vi "Main VI.vi"() -> ()   [LabVIEW 2016, in "Drona basic.lvlib"]
doc: "This VI performs the operation of basic drona, getting the active VI, populating the right click of control with Drona and also getting the drona path of the value changed control"
uses:
  Drona basic.lvlib
  Typedefs/Data.ctl
  <vilib>/SLL Toolkit/SLL Queued State Machine/Queue Driver/Typedefs/Queue Type.ctl
  Typedefs/cluster array.ctl
  <vilib>/Utility/miscctls.llb/LVPoint32TypeDef.ctl
  <vilib>/SLL Toolkit/SLL Queued State Machine/Queue Driver/Create Queue.vi
  <vilib>/SLL Toolkit/SLL Queued State Machine/Queue Driver/Enqueue an Item to Queue.vi
  <vilib>/SLL Toolkit/SLL Queued State Machine/Queue Driver/Dequeue Queue.vi
  <vilib>/SLL Toolkit/SLL Queued State Machine/Queue Driver/Enqueue N Items.vi
  <vilib>/SLL Toolkit/SLL Queued State Machine/Queue Driver/Flush Queue.vi
  <vilib>/SLL Toolkit/SLL Queued State Machine/Queue Driver/Release Queue.vi
  <vilib>/SLL Toolkit/SLL Queued State Machine/SLL QSM.lvlib
panel:
  out "Event and Drona Path:":string
  out "Error Out":errorcluster
  in  "Error In":errorcluster
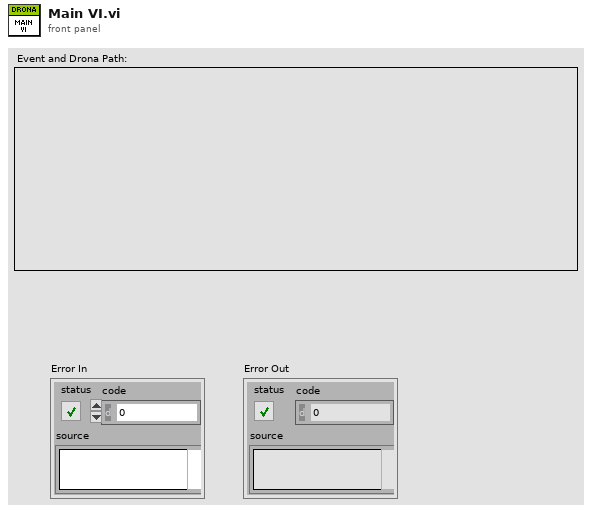
[diagram p1: front panel]
types:
  T1 = typedef "Drona basic.lvlib/Data.ctl" = cluster{"AppRef":refnum<vi>, "Active VIName":string, "Queue Ref":refnum<queue>, "ActiveVI reference":refnum<vi>, "Cluster references":refnum<vi>[], "Control References":refnum<vi>[], "Drona path,ref":T2[], "SelList ":refnum<vi>[], "Drona name":string, "Panes event refnum":refnum<event-registration>, "MenuRef":refnum<k9>, "Controls event refnum":refnum<event-registration>, "CtlRef":refnum<vi>, "Control name":string, "NewVal":variant, "OldVal":variant, "Point32":T3, "Ref array":refnum<vi>[], "Event ":string, "Event Registration Refnum ":refnum<event-registration>, "Subpanel reference":refnum<vi>, "Inserted VI ref":refnum<vi>, "SP Ref array":refnum<vi>[], "SP Registration Refnum":refnum<event-registration>, "User Events":cluster{"Panes event refnum":refnum<event-registration>, "Event Registration Refnum ":refnum<event-registration>, "SP Registration Refnum":refnum<event-registration>}}
  T2 = typedef "Drona basic.lvlib/cluster array.ctl" = cluster{"Control name":string, "Control reference":refnum<vi>}
  T3 = typedef "LVPoint32TypeDef.ctl" = cluster{"Horizontal":i32, "Vertical":i32}
  T4 = cluster{"Panes event refnum":refnum<event-registration>, "Event Registration Refnum ":refnum<event-registration>, "SP Registration Refnum":refnum<event-registration>}
  T5 = enum32{"Bad", "Idle", "Run top level", "Running"}
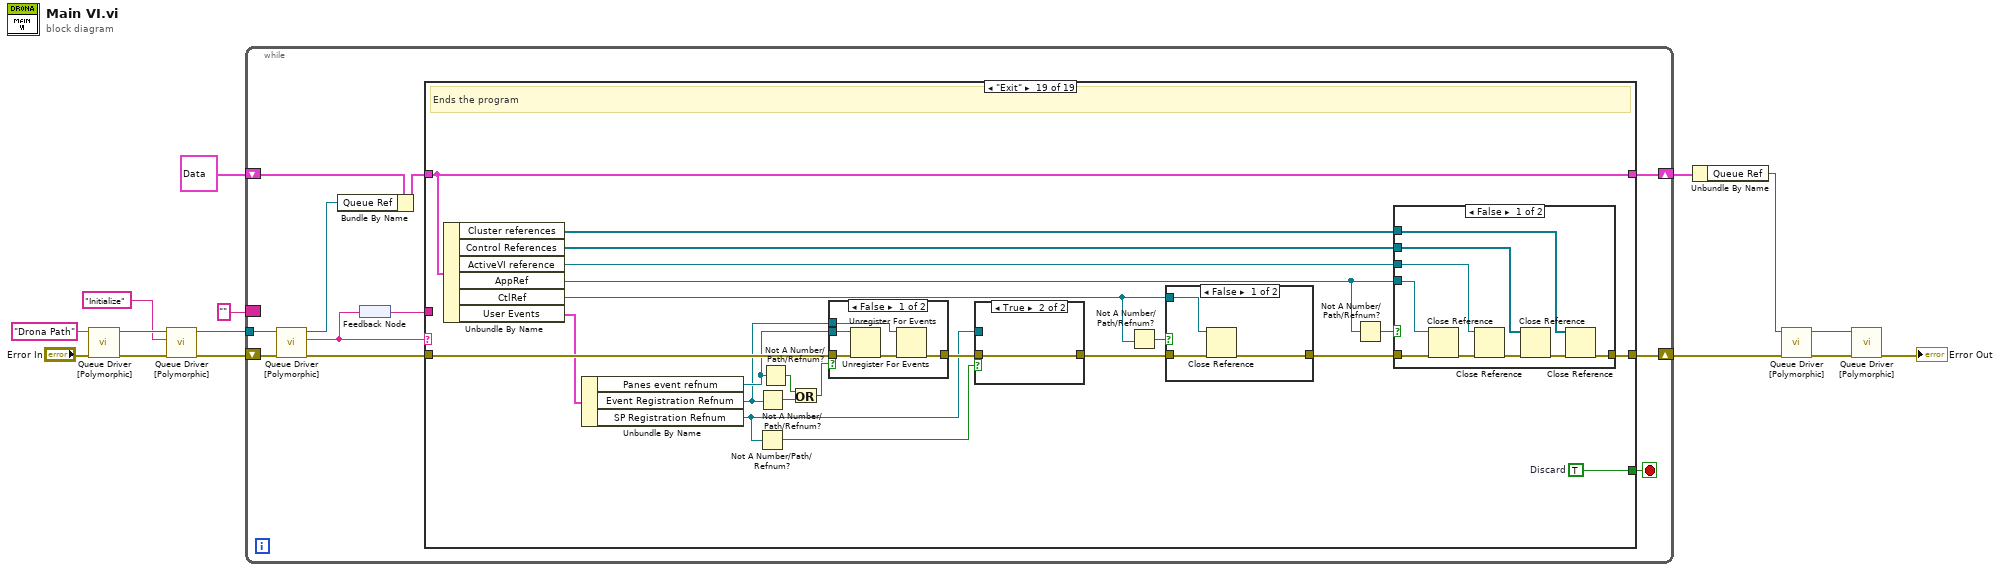
[diagram p0: block diagram]
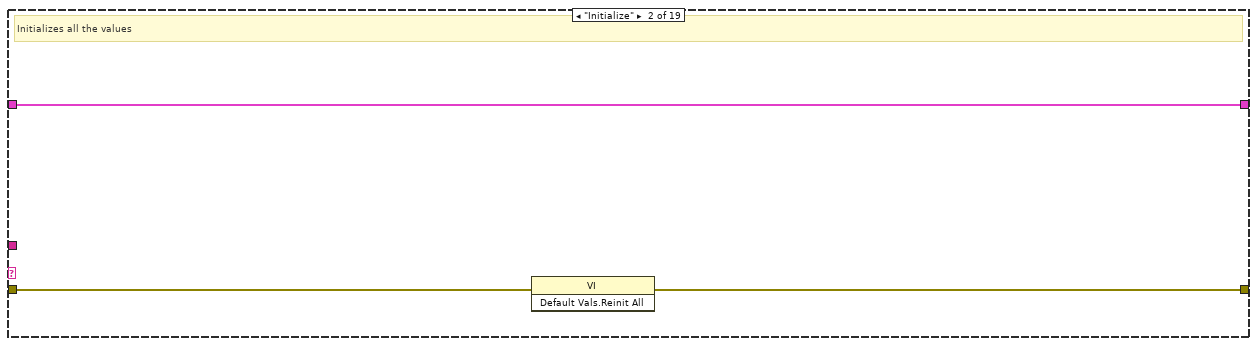
[diagram p3: hidden frame]
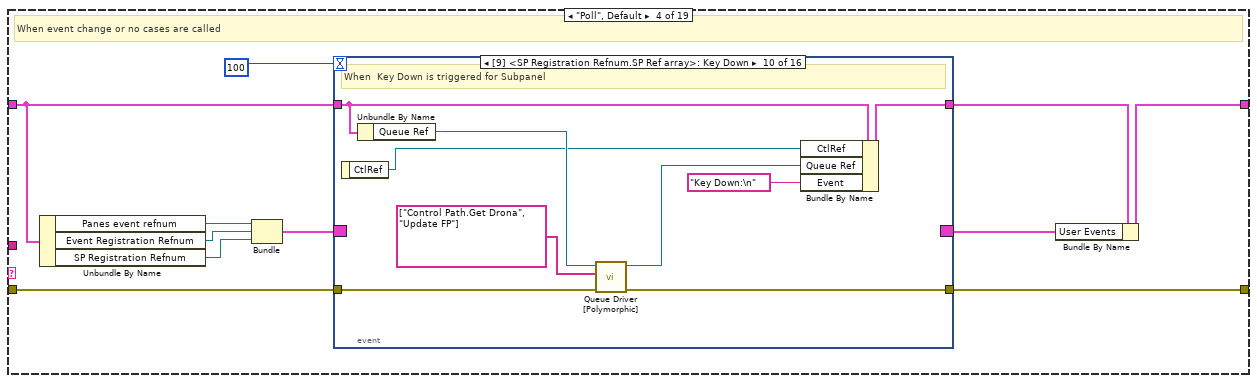
[diagram p5: hidden frame]
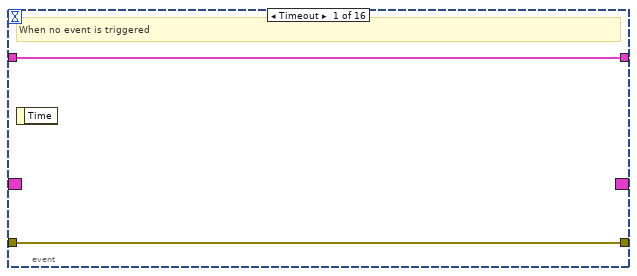
[diagram p6: hidden frame]
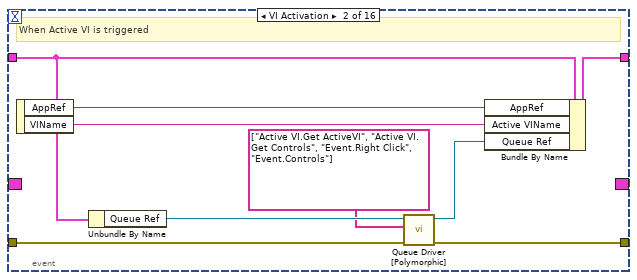
[diagram p7: hidden frame]
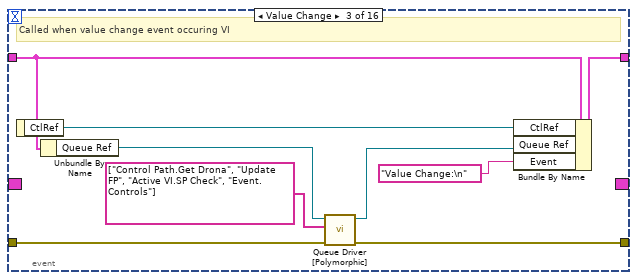
[diagram p8: hidden frame]
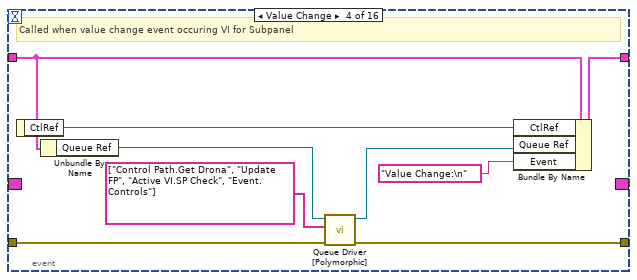
[diagram p9: hidden frame]
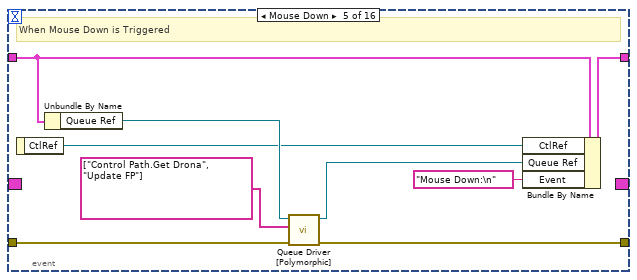
[diagram p10: hidden frame]
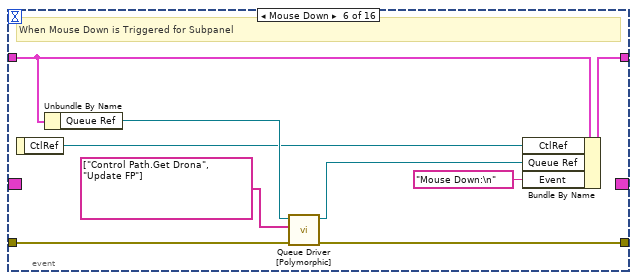
[diagram p11: hidden frame]
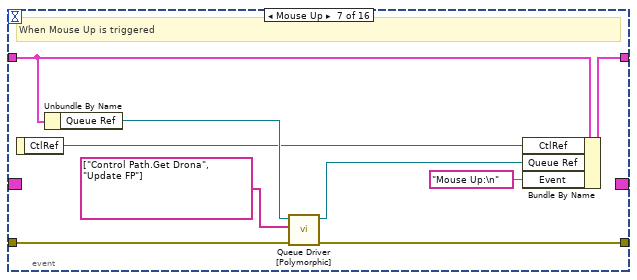
[diagram p12: hidden frame]
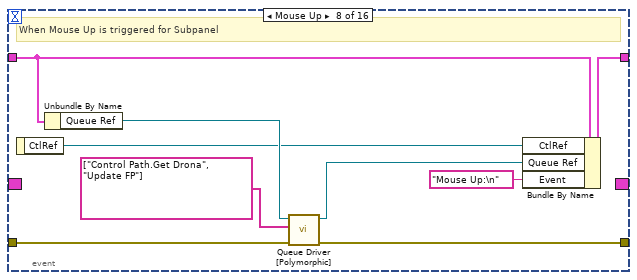
[diagram p13: hidden frame]
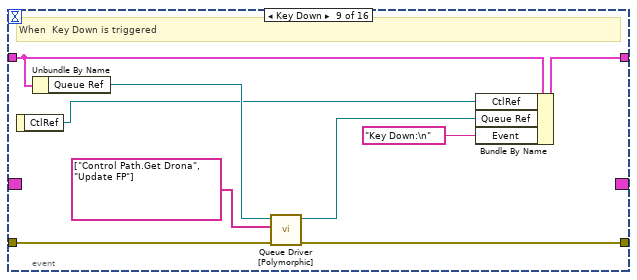
[diagram p14: hidden frame]
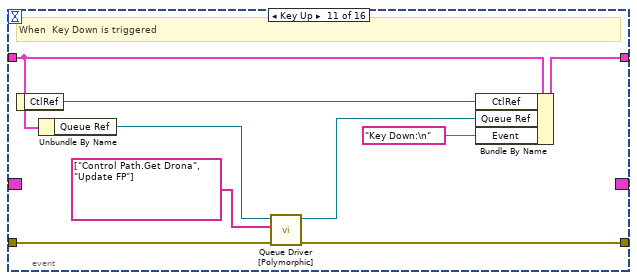
[diagram p15: hidden frame]
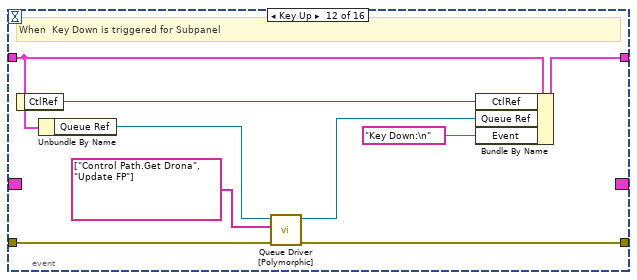
[diagram p16: hidden frame]
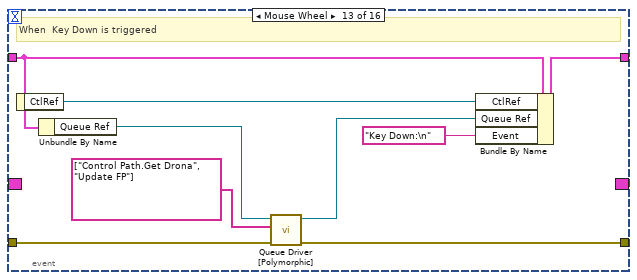
[diagram p17: hidden frame]
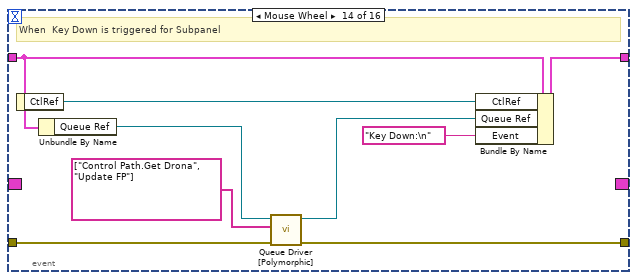
[diagram p18: hidden frame]
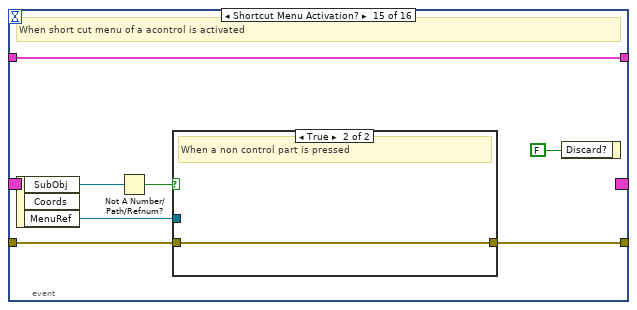
[diagram p19: hidden frame]
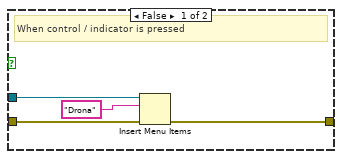
[diagram p20: hidden frame]
diagram:
  n1 = call-poly <vilib>:"Queue Driver [Polymorphic].vi"("Error In"="Error In", "Queue Name (Optional)"="Drona Path") -> ("Error Out"=w14:errorcluster, "Queue Ref"=w12:refnum<queue>)  [unwired: 8 in]
  n2 = call-poly <vilib>:"Queue Driver [Polymorphic].vi"("Error In"=w14, "Item to Add"="Initialize", "Queue Ref In"=w12) -> ("Error Out"=w9:errorcluster, "Queue Ref Out"=w8:refnum<queue>)  [unwired: 7 in]
  n3 = while {
    shift-right: [w26] -> w6
    shift-left: T1 {"AppRef"=refnum, "Active VIName"="", "Queue Ref"=refnum, "ActiveVI reference"=refnum, "Cluster references"=[], "Control References"=[], "Drona path,ref"=[], "SelList "=[], "Drona name"="", "Panes event refnum"=refnum, "MenuRef"=refnum, "Controls event refnum"=refnum, "CtlRef"=refnum, "Control name"="", "NewVal"=variant, "OldVal"=variant, "Point32"={"Horizontal"=0, "Vertical"=0}, "Ref array"=[], "Event "="", "Event Registration Refnum "=refnum, "Subpanel reference"=refnum, "Inserted VI ref"=refnum, "SP Ref array"=[], "SP Registration Refnum"=refnum, "User Events"={"Panes event refnum"=refnum, "Event Registration Refnum "=refnum, "SP Registration Refnum"=refnum}} -> [w23]
    tunnel: w8 -> [w24]
    shift-right: [w20] -> w7
    shift-left: w9 -> [w25]
    border: "" ("Feedback constant") -> [_]
    stop <- w18 stop-if-true
    n4 = call-poly <vilib>:"Queue Driver [Polymorphic].vi"("Error In"=w25, "Queue Ref In"=w24) -> ("Error Out"=w19:errorcluster, "Dequeue"=w17:string, "Queue Ref Out"=w21:refnum<queue>)  [unwired: 6 in, 1 out]
    n5 = Bundle By Name(cluster=w23, "Queue Ref"=w21) -> (w22:T1)
    n6 = feedback-in #1(w17) -> ()
    n7 = feedback #1() -> (w16:string)
    n8 = case shown="\"Exit\"" w17 {
      tunnel: [w28 w31 w33 w35 w185 w188 w190 w200 w221 w296 w319 w334 w356 w363 w370 w377 w380 w402 w423] -> w26
      tunnel: w22 -> [w28 w31 w33 w41 w185 w188 w190 w201 w222 w297 w319 w333 w356 w364 w371 w377 w381 w402 w423]
      tunnel: [w27 w29 w32 w43 w186 w187 w189 w191 w224 w302 w318 w330 w355 w365 w372 w376 w383 w401 w422] -> w20
      tunnel: w19 -> [w27 w30 w32 w42 w186 w187 w189 w203 w223 w303 w318 w326 w355 w360 w367 w376 w392 w401 w413]
      tunnel: [_ _ _ _ _ _ _ _ _ _ _ _ _ _ _ _ _ _ w424] -> w18
      tunnel: w16 -> [_ _ _ _ _ _ _ _ _ _ _ _ _ _ _ _ w389 _ _]
      frame "<-----------Initialize---------->" {
      }
      frame "Initialize" {
        # "Initializes all the values"
        n9 = invoke class="VI" method="Default Vals.Reinit All"(error in=w30) -> (error out=w29:errorcluster)  [unwired: 2 in, 2 out]
      }
      frame "<------Front panel cases------>" {
      }
      frame "Poll", Default {
        # "When event change or no cases are called"
        n10 = Unbundle By Name(w41) -> ("Panes event refnum"=w40:refnum<event-registration>, "Event Registration Refnum"=w37:refnum<event-registration>, "SP Registration Refnum"=w36:refnum<event-registration>)
        n11 = Bundle("Panes event refnum"=w40, "Event Registration Refnum"=w37, "SP Registration Refnum"=w36) -> (w39:T4)  [unwired: 1 in]
        n12 = event shown="[9] <SP Registration Refnum.SP Ref array>: Key Down" {
          selector: w39 -> [_ _ _ _ _ _ _ _ _ _ _ _ _ _ _ _]
          dyn-events: [_ _ _ _ _ _ _ _ _ _ _ _ _ _ _ _] -> w34
          timeout: 100 -> [_ _ _ _ _ _ _ _ _ _ _ _ _ _ _ _]
          tunnel: [w46 w55 w64 w73 w81 w90 w99 w108 w112 w121 w130 w139 w148 w157 w164 w178] -> w38
          tunnel: w41 -> [w46 w50 w61 w70 w80 w89 w98 w107 w111 w120 w129 w138 w147 w156 w164 w179]
          tunnel: [w45 w51 w62 w71 w79 w88 w97 w106 w118 w127 w136 w145 w154 w163 w169 w182] -> w43
          tunnel: w42 -> [w45 w52 w63 w72 w82 w91 w100 w109 w117 w126 w135 w144 w153 w162 w170 w176]
          event Timeout {
            # "When no event is triggered"
            n13 = event-data() -> ()  [unwired: 1 in, 1 out]
          }
          event VI Activation {
            # "When Active VI is triggered"
            n14 = event-data() -> ("AppRef"=w54:refnum<vi>, "VIName"=w53:string)  [unwired: 1 in]
            n15 = Unbundle By Name(w50) -> ("Queue Ref"=w49:refnum<queue>)
            n16 = call-poly <vilib>:"Queue Driver [Polymorphic].vi"("Error In"=w52, "Enqueue N"=string[] ["Active VI.Get ActiveVI", "Active VI.Get Controls", "Event.Right Click", "Event.Controls"], "Queue Ref In"=w49) -> ("Error Out"=w51:errorcluster, "Queue Ref Out"=w48:refnum<queue>)  [unwired: 7 in]
            n17 = Bundle By Name(cluster=w50, "AppRef"=w54, "Active VIName"=w53, "Queue Ref"=w48) -> (w55:T1)
          }
          event Value Change {
            # "Called when value change event occuring VI"
            n18 = event-data() -> ("CtlRef"=w58:refnum<vi>)  [unwired: 1 in]
            n19 = Unbundle By Name(w61) -> ("Queue Ref"=w60:refnum<queue>)
            n20 = call-poly <vilib>:"Queue Driver [Polymorphic].vi"("Error In"=w63, "Enqueue N"=string[] ["Control Path.Get Drona", "Update FP", "Active VI.SP Check", "Event.Controls"], "Queue Ref In"=w60) -> ("Error Out"=w62:errorcluster, "Queue Ref Out"=w59:refnum<queue>)  [unwired: 7 in]
            n21 = Bundle By Name(cluster=w61, "CtlRef"=w58, "Queue Ref"=w59, "Event"="Value Change:\n") -> (w64:T1)
          }
          event Value Change {
            # "Called when value change event occuring VI for Subpanel"
            n22 = event-data() -> ("CtlRef"=w67:refnum<vi>)  [unwired: 1 in]
            n23 = Unbundle By Name(w70) -> ("Queue Ref"=w69:refnum<queue>)
            n24 = call-poly <vilib>:"Queue Driver [Polymorphic].vi"("Error In"=w72, "Enqueue N"=string[] ["Control Path.Get Drona", "Update FP", "Active VI.SP Check", "Event.Controls"], "Queue Ref In"=w69) -> ("Error Out"=w71:errorcluster, "Queue Ref Out"=w68:refnum<queue>)  [unwired: 7 in]
            n25 = Bundle By Name(cluster=w70, "CtlRef"=w67, "Queue Ref"=w68, "Event"="Value Change:\n") -> (w73:T1)
          }
          event Mouse Down {
            # "When Mouse Down is Triggered"
            n26 = event-data() -> ("CtlRef"=w76:refnum<vi>)  [unwired: 1 in]
            n27 = Unbundle By Name(w80) -> ("Queue Ref"=w78:refnum<queue>)
            n28 = call-poly <vilib>:"Queue Driver [Polymorphic].vi"("Error In"=w82, "Enqueue N"=string[] ["Control Path.Get Drona", "Update FP"], "Queue Ref In"=w78) -> ("Error Out"=w79:errorcluster, "Queue Ref Out"=w77:refnum<queue>)  [unwired: 7 in]
            n29 = Bundle By Name(cluster=w80, "CtlRef"=w76, "Queue Ref"=w77, "Event"="Mouse Down:\n") -> (w81:T1)
          }
          event Mouse Down {
            # "When Mouse Down is Triggered for Subpanel"
            n30 = event-data() -> ("CtlRef"=w85:refnum<vi>)  [unwired: 1 in]
            n31 = Unbundle By Name(w89) -> ("Queue Ref"=w87:refnum<queue>)
            n32 = call-poly <vilib>:"Queue Driver [Polymorphic].vi"("Error In"=w91, "Enqueue N"=string[] ["Control Path.Get Drona", "Update FP"], "Queue Ref In"=w87) -> ("Error Out"=w88:errorcluster, "Queue Ref Out"=w86:refnum<queue>)  [unwired: 7 in]
            n33 = Bundle By Name(cluster=w89, "CtlRef"=w85, "Queue Ref"=w86, "Event"="Mouse Down:\n") -> (w90:T1)
          }
          event Mouse Up {
            # "When Mouse Up is triggered"
            n34 = event-data() -> ("CtlRef"=w94:refnum<vi>)  [unwired: 1 in]
            n35 = Unbundle By Name(w98) -> ("Queue Ref"=w96:refnum<queue>)
            n36 = call-poly <vilib>:"Queue Driver [Polymorphic].vi"("Error In"=w100, "Enqueue N"=string[] ["Control Path.Get Drona", "Update FP"], "Queue Ref In"=w96) -> ("Error Out"=w97:errorcluster, "Queue Ref Out"=w95:refnum<queue>)  [unwired: 7 in]
            n37 = Bundle By Name(cluster=w98, "CtlRef"=w94, "Queue Ref"=w95, "Event"="Mouse Up:\n") -> (w99:T1)
          }
          event Mouse Up {
            # "When Mouse Up is triggered for Subpanel"
            n38 = event-data() -> ("CtlRef"=w103:refnum<vi>)  [unwired: 1 in]
            n39 = Unbundle By Name(w107) -> ("Queue Ref"=w105:refnum<queue>)
            n40 = call-poly <vilib>:"Queue Driver [Polymorphic].vi"("Error In"=w109, "Enqueue N"=string[] ["Control Path.Get Drona", "Update FP"], "Queue Ref In"=w105) -> ("Error Out"=w106:errorcluster, "Queue Ref Out"=w104:refnum<queue>)  [unwired: 7 in]
            n41 = Bundle By Name(cluster=w107, "CtlRef"=w103, "Queue Ref"=w104, "Event"="Mouse Up:\n") -> (w108:T1)
          }
          event Key Down {
            # "When  Key Down is triggered"
            n42 = event-data() -> ("CtlRef"=w114:refnum<vi>)  [unwired: 1 in]
            n43 = Unbundle By Name(w111) -> ("Queue Ref"=w116:refnum<queue>)
            n44 = call-poly <vilib>:"Queue Driver [Polymorphic].vi"("Error In"=w117, "Enqueue N"=string[] ["Control Path.Get Drona", "Update FP"], "Queue Ref In"=w116) -> ("Error Out"=w118:errorcluster, "Queue Ref Out"=w113:refnum<queue>)  [unwired: 7 in]
            n45 = Bundle By Name(cluster=w111, "CtlRef"=w114, "Queue Ref"=w113, "Event"="Key Down:\n") -> (w112:T1)
          }
          event Key Down {
            # "When  Key Down is triggered for Subpanel"
            n46 = event-data() -> ("CtlRef"=w123:refnum<vi>)  [unwired: 1 in]
            n47 = Unbundle By Name(w120) -> ("Queue Ref"=w125:refnum<queue>)
            n48 = call-poly <vilib>:"Queue Driver [Polymorphic].vi"("Error In"=w126, "Enqueue N"=string[] ["Control Path.Get Drona", "Update FP"], "Queue Ref In"=w125) -> ("Error Out"=w127:errorcluster, "Queue Ref Out"=w122:refnum<queue>)  [unwired: 7 in]
            n49 = Bundle By Name(cluster=w120, "CtlRef"=w123, "Queue Ref"=w122, "Event"="Key Down:\n") -> (w121:T1)
          }
          event Key Up {
            # "When  Key Down is triggered"
            n50 = event-data() -> ("CtlRef"=w132:refnum<vi>)  [unwired: 1 in]
            n51 = Unbundle By Name(w129) -> ("Queue Ref"=w134:refnum<queue>)
            n52 = call-poly <vilib>:"Queue Driver [Polymorphic].vi"("Error In"=w135, "Enqueue N"=string[] ["Control Path.Get Drona", "Update FP"], "Queue Ref In"=w134) -> ("Error Out"=w136:errorcluster, "Queue Ref Out"=w131:refnum<queue>)  [unwired: 7 in]
            n53 = Bundle By Name(cluster=w129, "CtlRef"=w132, "Queue Ref"=w131, "Event"="Key Down:\n") -> (w130:T1)
          }
          event Key Up {
            # "When  Key Down is triggered for Subpanel"
            n54 = event-data() -> ("CtlRef"=w141:refnum<vi>)  [unwired: 1 in]
            n55 = Unbundle By Name(w138) -> ("Queue Ref"=w143:refnum<queue>)
            n56 = call-poly <vilib>:"Queue Driver [Polymorphic].vi"("Error In"=w144, "Enqueue N"=string[] ["Control Path.Get Drona", "Update FP"], "Queue Ref In"=w143) -> ("Error Out"=w145:errorcluster, "Queue Ref Out"=w140:refnum<queue>)  [unwired: 7 in]
            n57 = Bundle By Name(cluster=w138, "CtlRef"=w141, "Queue Ref"=w140, "Event"="Key Down:\n") -> (w139:T1)
          }
          event Mouse Wheel {
            # "When  Key Down is triggered"
            n58 = event-data() -> ("CtlRef"=w150:refnum<vi>)  [unwired: 1 in]
            n59 = Unbundle By Name(w147) -> ("Queue Ref"=w152:refnum<queue>)
            n60 = call-poly <vilib>:"Queue Driver [Polymorphic].vi"("Error In"=w153, "Enqueue N"=string[] ["Control Path.Get Drona", "Update FP"], "Queue Ref In"=w152) -> ("Error Out"=w154:errorcluster, "Queue Ref Out"=w149:refnum<queue>)  [unwired: 7 in]
            n61 = Bundle By Name(cluster=w147, "CtlRef"=w150, "Queue Ref"=w149, "Event"="Key Down:\n") -> (w148:T1)
          }
          event Mouse Wheel {
            # "When  Key Down is triggered for Subpanel"
            n62 = event-data() -> ("CtlRef"=w159:refnum<vi>)  [unwired: 1 in]
            n63 = Unbundle By Name(w156) -> ("Queue Ref"=w161:refnum<queue>)
            n64 = call-poly <vilib>:"Queue Driver [Polymorphic].vi"("Error In"=w162, "Enqueue N"=string[] ["Control Path.Get Drona", "Update FP"], "Queue Ref In"=w161) -> ("Error Out"=w163:errorcluster, "Queue Ref Out"=w158:refnum<queue>)  [unwired: 7 in]
            n65 = Bundle By Name(cluster=w156, "CtlRef"=w159, "Queue Ref"=w158, "Event"="Key Down:\n") -> (w157:T1)
          }
          event Shortcut Menu Activation? {
            # "When short cut menu of a acontrol is activated"
            n66 = event-data() -> ("SubObj"=w167:refnum<vi>, "MenuRef"=w165:refnum<k9>)  [unwired: 1 in, 1 out]
            n67 = Not A Number/Path/Refnum?(number/path/refnum=w167) -> (NaN/Path/Refnum?=w166:bool)
            n68 = case shown="True" w166 {
              tunnel: w170 -> [w174 w175]
              tunnel: [w173 w175] -> w169
              tunnel: w165 -> [w172 _]
              frame False {
                # "When control / indicator is pressed"
                n69 = Insert Menu Items(6:w174, 8:"Drona" ("item names"), 9:w172) -> (0:w173:errorcluster)  [unwired: 3 in, 2 out]
              }
              frame True {
                # "When a non control part is pressed"
              }
            }
            n70 = event-data("Discard?"=FALSE) -> ()  [unwired: 1 in, 1 out]
          }
          event Panel Close? {
            # "When panel close is pressed"
            n71 = event-data() -> ()  [unwired: 1 in, 2 out]
            n72 = Unbundle By Name(w179) -> ("Queue Ref"=w180:refnum<queue>)
            n73 = call-poly <vilib>:"Queue Driver [Polymorphic].vi"("Error In"=w176, "Item to Add"="Exit", "Queue Ref In"=w180) -> ("Error Out"=w182:errorcluster, "Queue Ref Out"=w177:refnum<queue>)  [unwired: 7 in]
            n74 = Bundle By Name(cluster=w179, "Queue Ref"=w177) -> (w178:T1)
            n75 = event-data("Discard?"=TRUE) -> ()  [unwired: 1 in, 1 out]
          }
        }
        n76 = Bundle By Name(cluster=w38, "User Events"=w34) -> (w35:T1)
      }
      frame "Update FP" {
        # "Updates the values to the front panel"
        n77 = Unbundle By Name(w185) -> ("Control name"=→"Event and Drona Path:":string)
      }
      frame "<-----Functional Cases------->" {
      }
      frame "<----------Active VI---------->" {
      }
      frame "Active VI.Get ActiveVI" {
        # "Gets the active vi's reference"
        n78 = Unbundle By Name(w201) -> ("AppRef"=w202:refnum<vi>, "Active VIName"=w199:string)
        n79 = Open VI Reference(application reference (local)=w202, vi path=w199, error in (no error)=w203) -> (vi reference=w193:refnum<vi>, error out=w194:errorcluster)  [unwired: 3 in]
        n80 = property class="VI"(reference=w193, error in=w194) -> (reference out=w195:refnum<vi>, error out=w197:errorcluster, "Exec.State"=w196:T5)
        n81 = case shown="\"Bad\", Default" w196 {
          tunnel: [errorcluster {"status"=TRUE, "code"=0, "source"="VI contains \nerrors to be \nexecuted "} ("error out") w209 w212 w213] -> w191
          tunnel: w197 -> [_ w210 w212 w213]
          tunnel: w195 -> [w204 w208 w211 w214]
          tunnel: [w204 w206 w211 w214] -> w192
          frame "Bad", Default {
          }
          frame "Idle" {
            w207 = FALSE ("Wait Until Done")
            n82 = invoke class="VI" method="Run VI"(reference=w208, error in=w210, "Wait until done"=w207, "Auto Dispose Ref"=w207) -> (reference out=w206:refnum<vi>, error out=w209:errorcluster)  [unwired: 1 in, 3 out]
          }
          frame "Run top level" {
          }
          frame "Running" {
          }
        }
        n83 = Bundle By Name(cluster=w201, "ActiveVI reference"=w192, "Ref array"=refnum<vi>[] []) -> (w200:T1)
      }
      frame "Active VI.Get Controls" {
        w217 = refnum<vi> refnum  # SubPanel
        # "Gets al the control's reference present in the active VI"
        n84 = Unbundle By Name(w222) -> ("SP Ref array"=w216:refnum<vi>[], "Ref array"=w226:refnum<vi>[], "ActiveVI reference"=w229:refnum<vi>)
        n85 = property class="VI"(reference=w229, error in=w223) -> (error out=w231:errorcluster, "Panel"=w230:refnum<vi>)  [unwired: 1 out]
        n86 = property class="Pnl"(reference=w230, error in=w231) -> (error out=w228:errorcluster, "Controls[]"=w227:refnum<vi>[])  [unwired: 1 out]
        n87 = for {
          shift-right: [w245] -> w224
          shift-left: w228 -> [w244]
          tunnel: w227 -> [w242] mode=indexing
          shift-right: [w238] -> w225
          shift-left: w226 -> [w240]
          shift-right: [w237] -> w220
          shift-left: refnum<vi> refnum ("InsertedVI") -> [w236]
          shift-right: [w235] -> w219
          shift-left: w217 -> [w234]
          shift-right: [w232] -> w215
          shift-left: w216 -> [w233]
          # "To get every controls"
          n88 = property class="Ctl"(reference=w242, error in=w244) -> (reference out=w239:refnum<vi>, error out=w243:errorcluster, "ClassName"=w241:string)
          n89 = case shown="\"Cluster\"" w241 {
            tunnel: [w252 w269 w283 w289] -> w245
            tunnel: w243 -> [w252 w265 w282 w294]
            tunnel: w240 -> [w251 w268 w281 w286]
            tunnel: w239 -> [w249 w267 w279 w292]
            tunnel: [w250 w263 w280 w286] -> w238
            tunnel: [w248 w257 w270 w288] -> w237
            tunnel: w236 -> [w248 w258 w275 _]
            tunnel: [w247 w255 w271 w287] -> w235
            tunnel: w234 -> [w247 w256 w272 _]
            tunnel: w233 -> [w246 w261 w278 w285]
            tunnel: [w246 w260 w277 w284] -> w232
            frame Default {
              # "For controls other thant cluster and tab"
              n90 = Insert Into Array(array=w251, new element=w249) -> (w250:refnum<vi>[])  [unwired: 1 in]
            }
            frame "Cluster" {
              w264 = refnum<vi> refnum  # Cluster
              # "If the control is a cluster"
              n91 = To More Specific Class(target class=w264, reference=w267, error in=w265) -> (specific class reference=w262:refnum<vi>, error out=w266:errorcluster)
              n92 = call "Mapping.vi"("Ref In"=w268, "SP Ref array in"=w261, "Clust Refnum"=w262, "error in (no error)"=w266) -> ("Ref Out"=w263:refnum<vi>[], "SP Ref array out"=w260:refnum<vi>[], "InsertedVI"=w254:refnum<vi>, "SubPnl Refnum"=w253:refnum<vi>, "error out"=w269:errorcluster)  [unwired: 7 in]
              n93 = Not A Number/Path/Refnum?(number/path/refnum=w254) -> (NaN/Path/Refnum?=w259:bool)
              n94 = Select(t=w258, s=w259, f=w254) -> (s? t:f=w257:refnum<vi>)
              n95 = Select(t=w256, s=w259, f=w253) -> (s? t:f=w255:refnum<vi>)
            }
            frame "TabControl" {
              # "If the control is a tab"
              n96 = call "TabControl.vi"("Ref In"=w281, "SP Ref array in"=w278, "Ctl Refnum"=w279, "error in (no error)"=w282) -> ("Ref Out"=w280:refnum<vi>[], "SP Ref array out"=w277:refnum<vi>[], "InsertedVI"=w274:refnum<vi>, "SubPnl Refnum"=w273:refnum<vi>, "error out"=w283:errorcluster)  [unwired: 7 in]
              n97 = Not A Number/Path/Refnum?(number/path/refnum=w274) -> (NaN/Path/Refnum?=w276:bool)
              n98 = Select(t=w275, s=w276, f=w274) -> (s? t:f=w270:refnum<vi>)
              n99 = Select(t=w272, s=w276, f=w273) -> (s? t:f=w271:refnum<vi>)
            }
            frame "SubPanel" {
              w291 = refnum<vi> refnum  # SubPanel
              n100 = To More Specific Class(target class=w291, reference=w292, error in=w294) -> (specific class reference=w287:refnum<vi>, error out=w293:errorcluster)
              n101 = property class="SubPnl"(reference=w287, error in=w293) -> (error out=w290:errorcluster, "InsertedVI"=w288:refnum<vi>)  [unwired: 1 out]
              n102 = call "SubPanel.vi"("Ref In"=w285, "VI reference"=w288, "error in (no error)"=w290) -> ("Ref Out"=w284:refnum<vi>[], "error out"=w289:errorcluster)  [unwired: 11 in]
            }
          }
        }
        n103 = Bundle By Name(cluster=w222, "SP Ref array"=w215, "Ref array"=w225, "Inserted VI ref"=w220, "Subpanel reference"=w219) -> (w221:T1)
      }
      frame "Active VI.SP Check" {
        # "This VI checks for if the inserted vi of subpanel is changed"
        n104 = Unbundle By Name(w297) -> ("Queue Ref"=w298:refnum<queue>, "Inserted VI ref"=w299:refnum<vi>, "Subpanel reference"=w300:refnum<vi>)
        n105 = Not A Number/Path/Refnum?(number/path/refnum=w300) -> (NaN/Path/Refnum?=w301:bool)
        n106 = case shown="False" w301 {
          tunnel: w303 -> [w315 w317]
          tunnel: [w310 w317] -> w302
          tunnel: w300 -> [w314 _]
          tunnel: w299 -> [w313 _]
          tunnel: w298 -> [w308 w316]
          tunnel: [w307 w316] -> w295
          frame False {
            # "When there is a subpanel"
            n107 = property class="SubPnl"(reference=w314, error in=w315) -> (error out=w311:errorcluster, "InsertedVI"=w312:refnum<vi>)  [unwired: 1 out]
            n108 = Not Equal?(x=w313, y=w312) -> (x != y?=w309:bool)
            n109 = Select(t=string[] ["Active VI.Get Controls ", "Event.Controls", "Event.Right Click"] ("Enqueue N"), s=w309, f=string[] [] ("Enqueue N")) -> (s? t:f=w304:string[])
            n110 = call-poly <vilib>:"Queue Driver [Polymorphic].vi"("Error In"=w311, "Enqueue N"=w304, "Queue Ref In"=w308) -> ("Error Out"=w310:errorcluster, "Queue Ref Out"=w307:refnum<queue>)  [unwired: 7 in]
          }
          frame True {
            # "When there is no subpanel"
          }
        }
        n111 = Bundle By Name(cluster=w297, "Queue Ref"=w295) -> (w296:T1)
      }
      frame "<-------Control Path--------->" {
      }
      frame "Control Path.Get Drona" {
        # "Gives out the Drona Path of the selected control"
        n112 = Unbundle By Name(w333) -> ("Event"=w332:string, "Subpanel reference"=w322:refnum<vi>, "Inserted VI ref"=w321:refnum<vi>, "CtlRef"=w320:refnum<vi>, "SP Ref array"=w331:refnum<vi>[])
        n113 = for {
          tunnel: w331 -> [w353] mode=indexing
          tunnel: w320 -> [w354]
          tunnel: [w352] -> w329
          shift-right: [w351] -> w325
          shift-left: w326 -> [w351]
          stop <- w352 stop-if-true
          n114 = Equal?(x=w354, y=w353) -> (x = y?=w352:bool)
        }
        n115 = call "Get Path.vi"("Control ref"=w320, "error in (no error)"=w325) -> ("Drona Path"=w324:string, "error out"=w323:errorcluster)  [unwired: 12 in]
        n116 = case shown="True" w329 {
          tunnel: w323 -> [w336 w349]
          tunnel: [w336 w348] -> w330
          tunnel: w324 -> [w335 w341]
          tunnel: [w335 w339] -> w327
          tunnel: w321 -> [_ w345]
          tunnel: w322 -> [_ w344]
          frame False {
          }
          frame True {
            w350 = refnum<vi> refnum  # Control
            n117 = property class="VI"(reference=w345, error in=w349) -> (error out=w346:errorcluster, "Name"=w343:string)  [unwired: 1 out]
            n118 = To More Generic Class(target class=w350, reference=w344) -> (generic class reference=w347:refnum<vi>)
            n119 = Concatenate Strings(w343, ">>" ("string"), w341) -> (w337:string)
            n120 = call "Get Path.vi"("Control ref"=w347, "error in (no error)"=w346) -> ("Drona Path"=w338:string, "error out"=w348:errorcluster)  [unwired: 12 in]
            n121 = Concatenate Strings(w338, ">>" ("string"), w337) -> (w339:string)
          }
        }
        n122 = Concatenate Strings(w332, w327) -> (w328:string)
        n123 = Bundle By Name(cluster=w333, "Control name"=w328) -> (w334:T1)
      }
      frame "<-----------Event------------->" {
      }
      frame "Event.Controls" {
        # "Registers value change for controls of the active vi"
        n124 = Unbundle By Name(w364) -> ("Ref array"=w362:refnum<vi>[], "SP Ref array"=w358:refnum<vi>[])
        n125 = register-events(error in=w360, w358, w358, w358, w358, w358, w358) -> (reference out=w357:refnum<event-registration>, error out=w359:errorcluster)  [unwired: 1 in]
        n126 = register-events(error in=w359, w362, w362, w362, w362, w362, w362) -> (reference out=w361:refnum<event-registration>, error out=w365:errorcluster)  [unwired: 1 in]
        n127 = Bundle By Name(cluster=w364, "SP Registration Refnum"=w357, "Event Registration Refnum"=w361) -> (w363:T1)
      }
      frame "Event.Right Click" {
        # "Gets the reg event for right click for active VI"
        n128 = Unbundle By Name(w371) -> ("ActiveVI reference"=w366:refnum<vi>)
        n129 = property class="VI"(reference=w366, error in=w367) -> (error out=w375:errorcluster, "Panel"=w374:refnum<vi>)  [unwired: 1 out]
        n130 = property class="Pnl"(reference=w374, error in=w375) -> (error out=w373:errorcluster, "Panes[]"=w368:refnum<vi>[])  [unwired: 1 out]
        n131 = register-events(error in=w373, w368) -> (reference out=w369:refnum<event-registration>, error out=w372:errorcluster)  [unwired: 1 in]
        n132 = Bundle By Name(cluster=w371, "Panes event refnum"=w369) -> (w370:T1)
      }
      frame "<--------Error Handling------>" {
      }
      frame "Error" {
        # "When error occurs, this case is called"
        n133 = Unbundle By Name(w381) -> ("Queue Ref"=w379:refnum<queue>)
        n134 = Unbundle By Name(w392) -> ("source"=w388:string)
        n135 = call <vilib>:"Clear Errors.vi"("error in (no error)"=w392) -> ("error out"=w393:errorcluster)  [unwired: 5 in, 1 out]
        n136 = Format Into String(format string="\\t%s \\n\n%s", initial string="Error Occured\nat", error in=w393, w389, w388) -> (resulting string=w387:string, error out=w382:errorcluster)
        n137 = Two Button Dialog(message=w387, 1:"Continue" ("F button name (\"Cancel\")"), 2:"Abort" ("T button name (\"OK\")")) -> (T button?=w384:bool)
        n138 = case shown="True" w384 {
          tunnel: [w395 w399] -> w383
          tunnel: w382 -> [w395 w400]
          tunnel: w379 -> [w394 w398]
          tunnel: [w394 w397] -> w378
          frame False {
            # "Continue"
          }
          frame True {
            # "Abort"
            n139 = call-poly <vilib>:"Queue Driver [Polymorphic].vi"("Error In"=w400, "Item to Add"="Exit", "Queue Ref In"=w398) -> ("Error Out"=w399:errorcluster, "Queue Ref Out"=w397:refnum<queue>)  [unwired: 7 in]
          }
        }
        n140 = Bundle By Name(cluster=w381, "Queue Ref"=w378) -> (w380:T1)
      }
      frame "<----------Exit case---------->" {
      }
      frame "Exit" {
        w424 = TRUE  # Discard
        # "Ends the program"
        n141 = Unbundle By Name(w423) -> ("Cluster references"=w419:refnum<vi>[], "Control References"=w420:refnum<vi>[], "ActiveVI reference"=w421:refnum<vi>, "AppRef"=w418:refnum<vi>, "CtlRef"=w414:refnum<vi>, "User Events"=w412:T4)
        n142 = Unbundle By Name(w412) -> ("Panes event refnum"=w408:refnum<event-registration>, "Event Registration Refnum"=w407:refnum<event-registration>, "SP Registration Refnum"=w403:refnum<event-registration>)
        n143 = Not A Number/Path/Refnum?(number/path/refnum=w403) -> (NaN/Path/Refnum?=w404:bool)
        n144 = Not A Number/Path/Refnum?(number/path/refnum=w407) -> (NaN/Path/Refnum?=w411:bool)
        n145 = Not A Number/Path/Refnum?(number/path/refnum=w408) -> (NaN/Path/Refnum?=w410:bool)
        n146 = Or(x=w410, y=w411) -> (x .or. y?=w409:bool)
        n147 = case shown="False" w409 {
          tunnel: w413 -> [w433 w434]
          tunnel: [w431 w434] -> w406
          tunnel: w408 -> [w430 _]
          tunnel: w407 -> [w429 _]
          frame False {
            n148 = Unregister For Events(event registration refnum=w430, error in=w433) -> (error out=w432:errorcluster)
            n149 = Unregister For Events(event registration refnum=w429, error in=w432) -> (error out=w431:errorcluster)
          }
          frame True {
          }
        }
        n150 = case shown="True" w404 {
          tunnel: w406 -> [w427 w428]
          tunnel: [w426 w428] -> w405
          tunnel: w403 -> [w425 _]
          frame False {
            n151 = Unregister For Events(event registration refnum=w425, error in=w427) -> (error out=w426:errorcluster)
          }
          frame True {
          }
        }
        n152 = Not A Number/Path/Refnum?(number/path/refnum=w414) -> (NaN/Path/Refnum?=w415:bool)
        n153 = case shown="False" w415 {
          tunnel: w405 -> [w437 w438]
          tunnel: [w436 w438] -> w416
          tunnel: w414 -> [w435 _]
          frame False {
            n154 = Close Reference(reference=w435, error in (no error)=w437) -> (error out=w436:errorcluster)
          }
          frame True {
          }
        }
        n155 = Not A Number/Path/Refnum?(number/path/refnum=w418) -> (NaN/Path/Refnum?=w417:bool)
        n156 = case shown="False" w417 {
          tunnel: w416 -> [w442 w448]
          tunnel: [w439 w448] -> w422
          tunnel: w421 -> [w447 _]
          tunnel: w420 -> [w444 _]
          tunnel: w419 -> [w443 _]
          tunnel: w418 -> [w440 _]
          frame False {
            n157 = Close Reference(reference=w440, error in (no error)=w442) -> (error out=w441:errorcluster)
            n158 = Close Reference(reference=w447, error in (no error)=w441) -> (error out=w445:errorcluster)
            n159 = Close Reference(reference=w444, error in (no error)=w445) -> (error out=w446:errorcluster)
            n160 = Close Reference(reference=w443, error in (no error)=w446) -> (error out=w439:errorcluster)
          }
          frame True {
          }
        }
      }
    }
  }
  n161 = Unbundle By Name(w6) -> ("Queue Ref"=w5:refnum<queue>)
  n162 = call-poly <vilib>:"Queue Driver [Polymorphic].vi"("Error In"=w7, "Queue Ref In"=w5) -> ("Error Out"=w4:errorcluster, "Queue Ref Out"=w3:refnum<queue>)  [unwired: 7 in, 1 out]
  n163 = call-poly <vilib>:"Queue Driver [Polymorphic].vi"("Error In"=w4, "Queue Ref In"=w3) -> ("Error Out"=→"Error Out":errorcluster)  [unwired: 9 in]
